vi "Secondary Page.vi"(8 "error in (no error)":errorcluster, 11 "Node Ptr":T1 format="%.0x") -> (0 "error out":errorcluster)   [LabVIEW 2020, in "AIM ARINC 664 System Explorer.lvlib" / "Implementation.lvlib"]
uses:
  Implementation.lvlib
  <vilib>/NI VeriStand/Custom Device API/Custom Device API.lvlib
  Scripting/AIM ARINC 664 Scripting.lvlib
  <vilib>/NI VeriStand/Custom Device API/Get Item Property (String).vi
  <vilib>/NI VeriStand/Custom Device API/Custom Device Item Ref.ctl
panel:
  in  "SHDocVw.IWebBrowser":refnum<k7>(container)
  in  "Property List":i32(listbox)
  in  "General Header":cluster{"Section Name":string}={"Section Name"="General Page Settings"}
  in  "Description":string
  out "Name":string
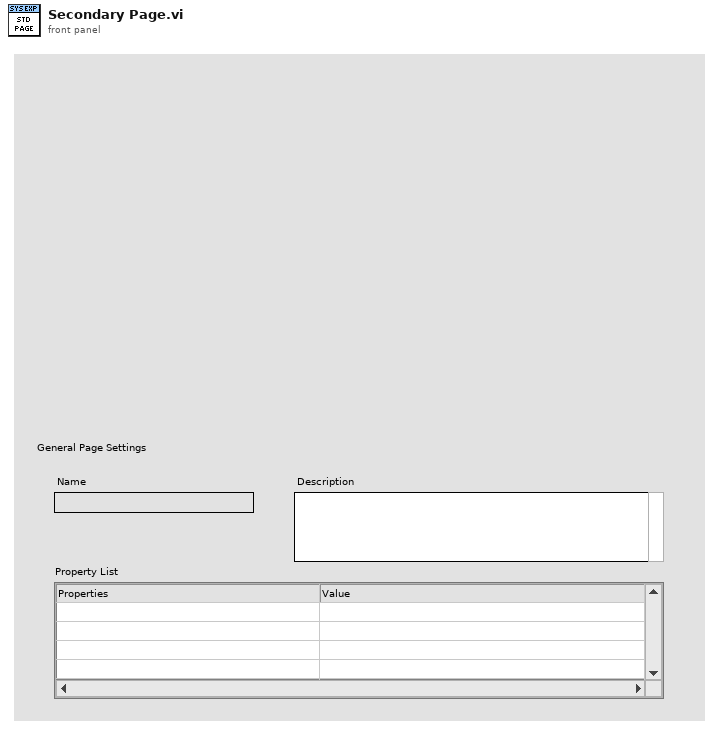
[diagram p1: front panel]
types:
  T1 = typedef "Custom Device API.lvlib/Custom Device Item Ref.ctl" = u64
  T2 = typedef "Custom Device API.lvlib/Custom Device Item Info.ctl" = cluster{"Name":string, "Is Channel":bool, "GUID":string, "Is Waveform":bool}
  T3 = typedef "Custom Device API.lvlib/Custom Device Commands.ctl" = enum16{"Default", "Item renamed", "Shutdown", "Dynamic button pressed"}
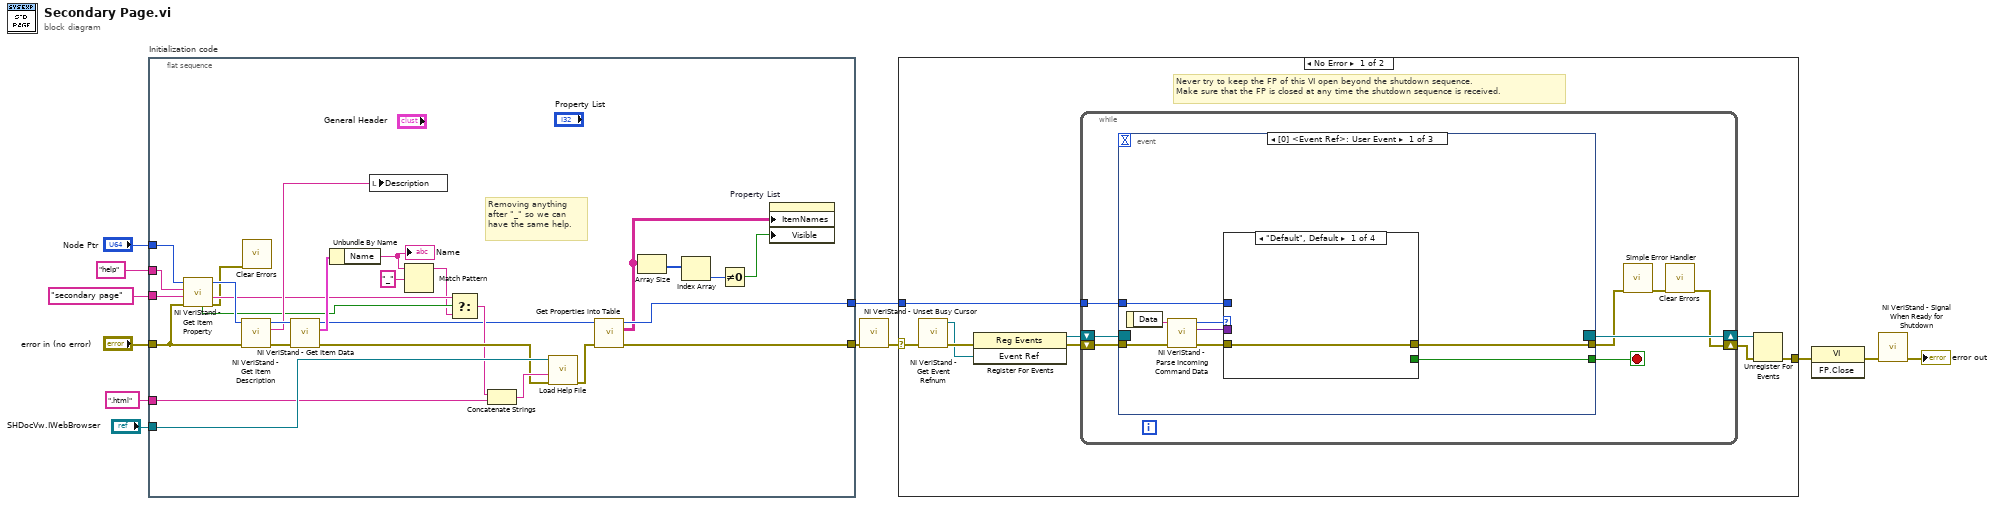
[diagram p0: block diagram]
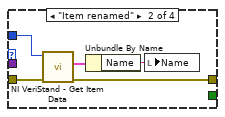
[diagram p2: hidden frame]
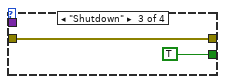
[diagram p3: hidden frame]
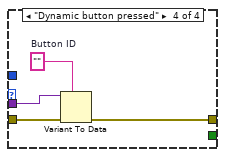
[diagram p4: hidden frame]
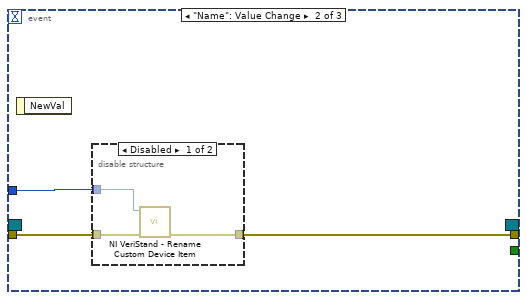
[diagram p5: hidden frame]
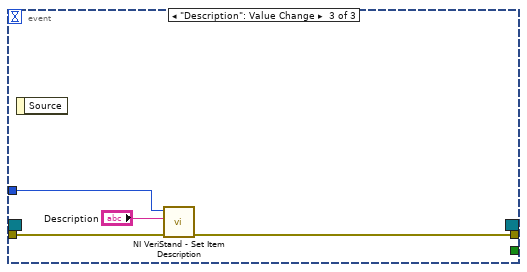
[diagram p7: hidden frame]
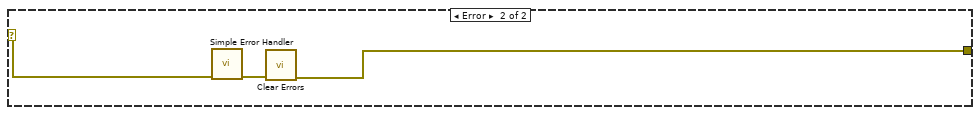
[diagram p8: hidden frame]
diagram:
  n1 = flat-sequence "Initialization code" {
    tunnel: "error in (no error)" -> [w25]
    tunnel: "Node Ptr" -> [w35]
    tunnel: [w18] -> w8
    tunnel: [w17] -> w5
    tunnel: "SHDocVw.IWebBrowser" -> [w36]
    tunnel: ".html" ("CD_CHM_Section") -> [w32]
    tunnel: "secondary page" ("Default Value") -> [w31]
    tunnel: "help" ("Property Name") -> [w29]
    frame #0 {
      # "Removing anything\nafter \"_\" so we can\nhave the same help."
      n2 = call-poly <vilib>:"NI VeriStand - Get Item Property.vi"("error in (no error)"=w25, "Default Value"=w31, "Property Name"=w29, "Item Ref in"=w35) -> ("error out"=w24:errorcluster, "Value"=w28:string, "Item Ref out"=w34:T1, "Found?"=w27:bool)  [unwired: 4 in]
      n3 = call <vilib>:"NI VeriStand - Get Item Description.vi"("error in (no error)"=w25, "Item Ref in"=w34) -> ("error out"=w39:errorcluster, "Description"=w37:string, "Item Ref out"=w40:T1)  [unwired: 7 out]
      n4 = call <vilib>:"Clear Errors.vi"("error in (no error)"=w24) -> ()  [unwired: 5 in, 2 out]
      n5 = call <vilib>:"NI VeriStand - Get Item Data.vi"("error in (no error)"=w39, "Item Ref in"=w40) -> ("error out"=w30:errorcluster, "Item Info"=w38:T2, "Item Ref out"=w20:T1)  [unwired: 7 out]
      n6 = Unbundle By Name(w38) -> ("Name"=w23:string)
      "Name" <- w23
      n7 = local write "Description"(w37) -> ()
      n8 = Match Pattern(string=w23, regular expression="_") -> (before substring=w21:string)  [unwired: 1 in, 3 out]
      n9 = Select(t=w28, s=w27, f=w21) -> (s? t:f=w26:string)
      n10 = Concatenate Strings(w26, w32) -> (w33:string)
      n11 = call "Load Help File.vi"("error in (no error)"=w30, "HTML File to Load"=w33, "Browser"=w36) -> ("error out"=w19:errorcluster)  [unwired: 8 in]
      n12 = call "Get Properties into Table.vi"("error in"=w19, "Item Ref in"=w20) -> ("error out"=w18:errorcluster, "Property Names"=w16:string[][], "Item Ref out"=w17:T1)  [unwired: 7 in]
      n13 = Array Size(array=w16) -> (size(s)=w14:i32[])
      n14 = Index Array(array=w14) -> (element=w13:i32)  [unwired: 1 in]
      n15 = Not Equal To 0?(x=w13) -> (x != 0?=w15:bool)
      n16 = property on="Property List" class="MCListbox (strict)"("ItemNames"=w16, "Visible"=w15) -> ()  [unwired: 2 in, 2 out]
    }
  }
  n17 = call <vilib>:"NI VeriStand - Unset Busy Cursor.vi"("error in (no error)"=w8) -> ("error out"=w7:errorcluster)  [unwired: 10 out]
  n18 = case shown="No Error" w7 {
    selector: w7 -> [w41 w91]
    tunnel: [w46 w89] -> w12
    tunnel: w5 -> [w42 _]
    frame No Error {
      # "Never try to keep the FP of this VI open beyond the shutdown sequence.\nMake sure that the FP is closed at any time the shutdown sequence is received."
      n19 = call <vilib>:"NI VeriStand - Get Event Refnum.vi"("error in (no error)"=w41) -> ("error out"=w49:errorcluster, "Event Ref"=w45:refnum<user-event>)  [unwired: 9 out]
      n20 = register-events(error in=w49, w45) -> (reference out=w43:refnum<event-registration>, error out=w44:errorcluster)  [unwired: 1 in]
      n21 = while {
        tunnel: w42 -> [w53]
        shift-right: [w50] -> w47
        shift-left: w44 -> [w56]
        shift-right: [w57] -> w48
        shift-left: w43 -> [w55]
        stop <- w54 stop-if-true
        n22 = event shown="[0] <Event Ref>: User Event" {
          selector: w55 -> [_ _ _]
          dyn-events: [_ _ _] -> w57
          timeout: _ -> [_ _ _]
          tunnel: w56 -> [w65 w80 w87]
          tunnel: [w61 _ _] -> w54
          tunnel: [w60 w79 w86] -> w52
          tunnel: w53 -> [w59 w78 w88]
          event User Event {
            n23 = event-data() -> ("Data"=w64:string)  [unwired: 1 out]
            n24 = call <vilib>:"NI VeriStand - Parse Incoming Command Data.vi"("error in (no error)"=w65, "Incoming data"=w64) -> ("error out"=w63:errorcluster, "Outgoing data"=w58:variant, "Action"=w62:T3)  [unwired: 7 out]
            n25 = case shown="\"Default\", Default" w62 {
              tunnel: w63 -> [w66 w71 w72 w77]
              tunnel: [_ _ TRUE _] -> w61
              tunnel: [w66 w68 w72 w74] -> w60
              tunnel: w59 -> [_ w70 _ _]
              tunnel: w58 -> [_ _ _ w76]
              frame "Default", Default {
              }
              frame "Item renamed" {
                n26 = call <vilib>:"NI VeriStand - Get Item Data.vi"("error in (no error)"=w71, "Item Ref in"=w70) -> ("error out"=w68:errorcluster, "Item Info"=w69:T2)  [unwired: 8 out]
                n27 = Unbundle By Name(w69) -> ("Name"=w67:string)
                n28 = local write "Name"(w67) -> ()
              }
              frame "Shutdown" {
              }
              frame "Dynamic button pressed" {
                w75 = ""  # Button ID
                n29 = Variant To Data(error in=w77, type=w75, Variant=w76) -> (error out=w74:errorcluster)  [unwired: 1 out]
              }
            }
          }
          event "Name": Value Change {
            n30 = event-data() -> ()  [unwired: 2 out]
            n31 = disable-structure shown="Disabled" {
              disable-tunnel: w80 -> [w83 w84]
              disable-tunnel: [w82 w84] -> w79
              disable-tunnel: w78 -> [w81 _]
              frame Disabled {
                n32 = call <vilib>:"NI VeriStand - Rename Custom Device Item.vi"("error in (no error)"=w83, "Item Ref in"=w81) -> ("error out"=w82:errorcluster)  [unwired: 2 in, 7 out]
              }
              frame Enabled {
              }
            }
          }
          event "Description": Value Change {
            n33 = event-data() -> ()  [unwired: 2 out]
            n34 = call <vilib>:"NI VeriStand - Set Item Description.vi"("error in (no error)"=w87, "Description"="Description", "Item Ref in"=w88) -> ("error out"=w86:errorcluster)  [unwired: 8 out]
          }
        }
        n35 = call <vilib>:"Simple Error Handler.vi"("error in (no error)"=w52) -> ("error out"=w51:errorcluster)  [unwired: 1 in, 7 out]
        n36 = call <vilib>:"Clear Errors.vi"("error in (no error)"=w51) -> ("error out"=w50:errorcluster)  [unwired: 1 in, 5 out]
      }
      n37 = Unregister For Events(event registration refnum=w48, error in=w47) -> (error out=w46:errorcluster)
    }
    frame Error {
      n38 = call <vilib>:"Simple Error Handler.vi"("error in (no error)"=w91) -> ("error out"=w90:errorcluster)  [unwired: 1 in, 7 out]
      n39 = call <vilib>:"Clear Errors.vi"("error in (no error)"=w90) -> ("error out"=w89:errorcluster)  [unwired: 1 in, 5 out]
    }
  }
  n40 = invoke class="VI" method="FP.Close"(error in=w12) -> (error out=w11:errorcluster)  [unwired: 2 in, 2 out]
  n41 = call <vilib>:"NI VeriStand - Signal When Ready for Shutdown.vi"("error in (no error)"=w11) -> ("error out"=→"error out":errorcluster)  [unwired: 10 out]
